vi "test_PlaceBottomvalidation.vi"(11 "Test Case In":refnum<class "RelativePlacingTests.lvclass">) -> (0 "error out":errorcluster, 3 "Test Case Out":refnum<class "RelativePlacingTests.lvclass">)   [LabVIEW 2023, in "RelativePlacingTests.lvclass"]
uses:
  RelativePlacingTests.lvclass
  C:/Program Files (x86)/National Instruments/LabVIEW 2023/vi.lib/Astemes/LUnit/Test Case.lvclass
  <vilib>/Astemes/LUnit/Test Case.lvclass/Test Case.ctl
  <vilib>/Astemes/LUnit/Core/LUnit Test Case/Private/Append Fail Result.vi
  <vilib>/Astemes/LUnit/Core/LUnit Test Case/Private/Append Pass Result.vi
  <vilib>/Astemes/LUnit/Core/LUnit Test Case/Private/Run In UI.vi
  <vilib>/Utility/error.llb/Clear Errors.vi
  RelativePlacingTests.lvclass/RelativePlacingTests.ctl
  <vilib>/Astemes/LUnit/Test Case.lvclass
  C:/Program Files (x86)/National Instruments/LabVIEW 2023/vi.lib/Astemes/LUnit/LUnit Runnable.lvclass
  C:/projects/TLC_Geometry/tests/RelativePlacingTests/RelativePlacingTests.lvclass
panel:
  in  "movingObject":string
  in  "anchor":dbl
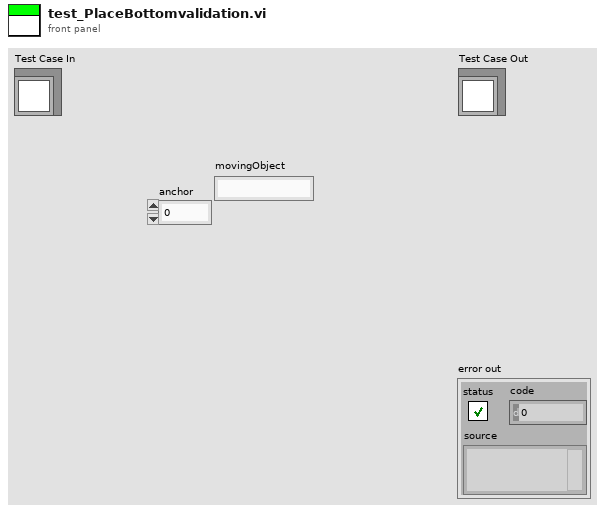
[diagram p1: front panel]
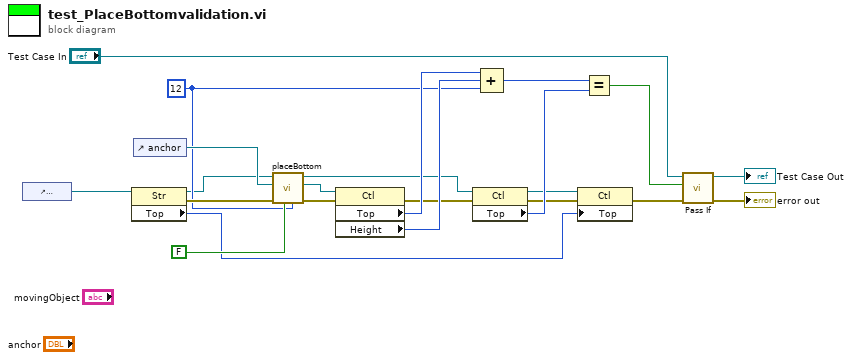
[diagram p0: block diagram]
diagram:
  w14 = u16 12 ("spacing")
  n1 = control-ref of="movingObject"() -> (w13:refnum<vi>)
  n2 = property class="Str"(reference=w13) -> (reference out=w12:refnum<vi>, error out=w17:errorcluster, "Top"=w8:i32)  [unwired: 1 in]
  n3 = control-ref of="anchor"() -> (w18:refnum<vi>)
  n4 = call "placeBottom.vi"("spacing[pixel]"=w14, "useControlBodyOnly"=FALSE, "error in (no error)"=w17, "anchorObject"=w18, "movingObject"=w12) -> ("error out"=w3:errorcluster, "anchorObject(dup)"=w6:refnum<vi>, "movingObject(dup)"=w5:refnum<vi>)  [unwired: 4 in]
  n5 = property class="Ctl"(reference=w6, error in=w3) -> (error out=w2:errorcluster, "Top"=w16:i32, "Height"=w15:u32)  [unwired: 1 out]
  n6 = property class="Ctl"(reference=w5, error in=w2) -> (reference out=w4:refnum<vi>, error out=w1:errorcluster, "Top"=w10:i32)
  n7 = Compound Arithmetic op=ADD(w16, w15, w14) -> (w11:u32)
  n8 = property class="Ctl"(reference=w4, error in=w1, "Top"=w8) -> (error out=w9:errorcluster)  [unwired: 1 out]
  n9 = Equal?(x=w11, y=w10) -> (x = y?=w7:bool)
  n10 = call <vilib>:"Pass If.vi"("error in (no error)"=w9, "Pass?"=w7, "LUnit Test Case In"="Test Case In") -> ("error out"=→"error out":errorcluster, "LUnit Test Case Out"=→"Test Case Out":refnum<class "RelativePlacingTests.lvclass">)  [unwired: 7 in]
